vi "RecursiveNavigateHCC.vi"(9 "SearchingFor":string="body", 11 "data":string="<!DOCTYPE HTML PUBLIC \"-//IETF//DTD HTML//EN\">\r\n<HTML>\r\n<HEAD>\r\n<meta name=\"generator\" content=\"Microsoft&reg; HTML Help Workshop 4.1\">\r\n<!-- Sitemap 1.0 -->\r\n</head>\r\n<body>\r\n   <OBJECT type=\"text/site properties\">\r\n     <param name=\"Window Styles\" value=\"0x800025\">\r\n     <param name=\"comment\" value=\"title:Online Help\">\r\n     <param name=\"comment\" value=\"base:index.htm\">\r\n   </OBJECT>\r\n   <UL>\r\n      <LI><OBJECT type=\"text/sitemap\">\r\n            <param name=\"Name\" value=\"Main\">\r\n            <param name=\"Local\" value=\"main/main.html\">\r\n            <param name=\"ImageNumber\" value=\"2\">\r\n          </OBJECT>\r\n      <LI><OBJECT type=\"text/sitemap\">\r\n            <param name=\"Name\" value=\"Alarms\">\r\n            <param name=\"Local\" value=\"alarms/alarms.html\">\r\n            <param name=\"ImageNumber\" value=\"11\">\r\n          </OBJECT>\r\n      <LI><OBJECT type=\"text/sitemap\">\r\n            <param name=\"Name\" value=\"Calibration\">\r\n            <param name=\"Local\" value=\"calibration/calibration.html\">\r\n            <param name=\"ImageNumber\" value=\"11\">\r\n          </OBJECT>\r\n      <LI><OBJECT type=\"text/sitemap\">\r\n            <param name=\"Name\" value=\"Channel setting\">\r\n            <param name=\"Local\" value=\"channels%20setting/channel_setting.html\">\r\n            <param name=\"ImageNumber\" value=\"11\">\r\n          </OBJECT>\r\n      <LI><OBJECT type=\"text/sitemap\">\r\n            <param name=\"Name\" value=\"Create deltas\">\r\n            <param name=\"Local\" value=\"create%20delta/create_deltas.html\">\r\n            <param name=\"ImageNumber\" value=\"11\">\r\n          </OBJECT>\r\n      <LI><OBJECT type=\"text/sitemap\">\r\n            <param name=\"Name\" value=\"Criteria window\">\r\n            <param name=\"Local\" value=\"criteria/criteria_window.html\">\r\n            <param name=\"ImageNumber\" value=\"11\">\r\n          </OBJECT>\r\n      <LI><OBJECT type=\"text/sitemap\">\r\n            <param name=\"Name\" value=\"Filters\">\r\n            <param name=\"Local\" value=\"filters/filters.html\">\r\n          </OBJECT>\r\n      <UL>\r\n         <LI><OBJECT type=\"text/sitemap\">\r\n               <param name=\"Name\" value=\"Differential\">\r\n               <param name=\"Local\" value=\"filters/differential_filter.html\">\r\n               <param name=\"ImageNumber\" value=\"11\">\r\n             </OBJECT>\r\n         <LI><OBJECT type=\"text/sitemap\">\r\n               <param name=\"Name\" value=\"IIR-FIR\">\r\n               <param name=\"Local\" value=\"filters/iir_fir_filter.html\">\r\n               <param name=\"ImageNumber\" value=\"11\">\r\n             </OBJECT>\r\n         <LI><OBJECT type=\"text/sitemap\">\r\n               <param name=\"Name\" value=\"Median\">\r\n               <param name=\"Local\" value=\"filters/median_filter.html\">\r\n               <param name=\"ImageNumber\" value=\"11\">\r\n             </OBJECT>\r\n         <LI><OBJECT type=\"text/sitemap\">\r\n               <param name=\"Name\" value=\"Wavelet\">\r\n               <param name=\"Local\" value=\"filters/wavelet_filter.html\">\r\n               <param name=\"ImageNumber\" value=\"11\">\r\n             </OBJECT>\r\n      </UL>\r\n      <LI><OBJECT type=\"text/sitemap\">\r\n            <param name=\"Name\" value=\"Last defect window\">\r\n            <param name=\"Local\" value=\"last%20defect%20window/last_defect_window.html\">\r\n            <param name=\"ImageNumber\" value=\"11\">\r\n          </OBJECT>\r\n      <LI><OBJECT type=\"text/sitemap\">\r\n            <param name=\"Name\" value=\"Live view\">\r\n            <param name=\"Local\" value=\"live%20view/live_view.html\">\r\n            <param name=\"ImageNumber\" value=\"11\">\r\n          </OBJECT>\r\n      <LI><OBJECT type=\"text/sitemap\">\r\n            <param name=\"Name\" value=\"Oscilloscope\">\r\n            <param name=\"Local\" value=\"oscilloscope/oscilloscope.html\">\r\n            <param name=\"ImageNumber\" value=\"11\">\r\n          </OBJECT>\r\n      <LI><OBJECT type=\"text/sitemap\">\r\n            <param name=\"Name\" value=\"Record data\">\r\n            <param name=\"Local\" value=\"record%20data/record_data_window.html\">\r\n            <param name=\"ImageNumber\" value=\"11\">\r\n          </OBJECT>\r\n      <LI><OBJECT type=\"text/sitemap\">\r\n            <param name=\"Name\" value=\"Stripchart\">\r\n            <param name=\"Local\" value=\"stripchart%20Vpp/stripchart.html\">\r\n            <param name=\"ImageNumber\" value=\"11\">\r\n          </OBJECT>\r\n      <LI><OBJECT type=\"text/sitemap\">\r\n            <param name=\"Name\" value=\"System info\">\r\n            <param name=\"Local\" value=\"system%20info/system_info.html\">\r\n            <param name=\"ImageNumber\" value=\"11\">\r\n          </OBJECT>\r\n      <LI><OBJECT type=\"text/sitemap\">\r\n            <param name=\"Name\" value=\"System settings\">\r\n            <param name=\"Local\" value=\"system%20settings/system_settings.html\">\r\n            <param name=\"ImageNumber\" value=\"11\">\r\n          </OBJECT>\r\n      <LI><OBJECT type=\"text/sitemap\">\r\n            <param name=\"Name\" value=\"Vumeter\">\r\n            <param name=\"Local\" value=\"vumeter/vumeter.html\">\r\n            <param name=\"ImageNumber\" value=\"11\">\r\n          </OBJECT>\r\n      <LI><OBJECT type=\"text/sitemap\">\r\n            <param name=\"Name\" value=\"Wizard\">\r\n            <param name=\"Local\" value=\"wizard/wizard.html\">\r\n          </OBJECT>\r\n      <UL>\r\n         <LI><OBJECT type=\"text/sitemap\">\r\n               <param name=\"Name\" value=\"Step 1\">\r\n               <param name=\"Local\" value=\"wizard/wizard_step_1.html\">\r\n               <param name=\"ImageNumber\" value=\"11\">\r\n             </OBJECT>\r\n         <LI><OBJECT type=\"text/sitemap\">\r\n               <param name=\"Name\" value=\"Step 2\">\r\n               <param name=\"Local\" value=\"wizard/wizard_step_2.html\">\r\n               <param name=\"ImageNumber\" value=\"11\">\r\n             </OBJECT>\r\n         <LI><OBJECT type=\"text/sitemap\">\r\n               <param name=\"Name\" value=\"Step 3\">\r\n               <param name=\"Local\" value=\"wizard/wizard_step_3.html\">\r\n               <param name=\"ImageNumber\" value=\"11\">\r\n             </OBJECT>\r\n         <LI><OBJECT type=\"text/sitemap\">\r\n               <param name=\"Name\" value=\"Step 4\">\r\n               <param name=\"Local\" value=\"wizard/wizard_step_4.html\">\r\n               <param name=\"ImageNumber\" value=\"11\">\r\n             </OBJECT>\r\n         <LI><OBJECT type=\"text/sitemap\">\r\n               <param name=\"Name\" value=\"Step 5\">\r\n               <param name=\"Local\" value=\"wizard/wizard_step_5.html\">\r\n               <param name=\"ImageNumber\" value=\"11\">\r\n             </OBJECT>\r\n         <LI><OBJECT type=\"text/sitemap\">\r\n               <param name=\"Name\" value=\"Step 6\">\r\n               <param name=\"Local\" value=\"wizard/wizard_step_6.html\">\r\n               <param name=\"ImageNumber\" value=\"11\">\r\n             </OBJECT>\r\n      </UL>\r\n   </UL>\r\n</BODY>\r\n</HTML>\r\n") -> (1 "ItemTags":string[](array[string]), 2 "Ident":i32[](array[numeric]), 3 "ItemNames":string[](array[string]))   [LabVIEW 2016, in "Folder_Mgmt.lvclass"]
uses:
  Folder_Mgmt.lvclass
  <vilib>/regexp/Match Regular Expression.xnode
panel:
  in  "TestString":string="<!DOCTYPE HTML PUBLIC \"-//IETF//DTD HTML//EN\">\r\n<HTML>\r\n<HEAD>\r\n<meta name=\"generator\" content=\"Microsoft&reg; HTML Help Workshop 4.1\">\r\n<!-- Sitemap 1.0 -->\r\n</head>\r\n<body>\r\n   <OBJECT type=\"text/site properties\">\r\n     <param name=\"Window Styles\" value=\"0x800025\">\r\n     <param name=\"comment\" value=\"title:Online Help\">\r\n     <param name=\"comment\" value=\"base:index.htm\">\r\n   </OBJECT>\r\n   <UL>\r\n      <LI><OBJECT type=\"text/sitemap\">\r\n            <param name=\"Name\" value=\"Main\">\r\n            <param name=\"Local\" value=\"main/main.html\">\r\n            <param name=\"ImageNumber\" value=\"2\">\r\n          </OBJECT>\r\n      <LI><OBJECT type=\"text/sitemap\">\r\n            <param name=\"Name\" value=\"Alarms\">\r\n            <param name=\"Local\" value=\"alarms/alarms.html\">\r\n            <param name=\"ImageNumber\" value=\"11\">\r\n          </OBJECT>\r\n   </UL>\r\n</BODY>\r\n</HTML>\r\n"
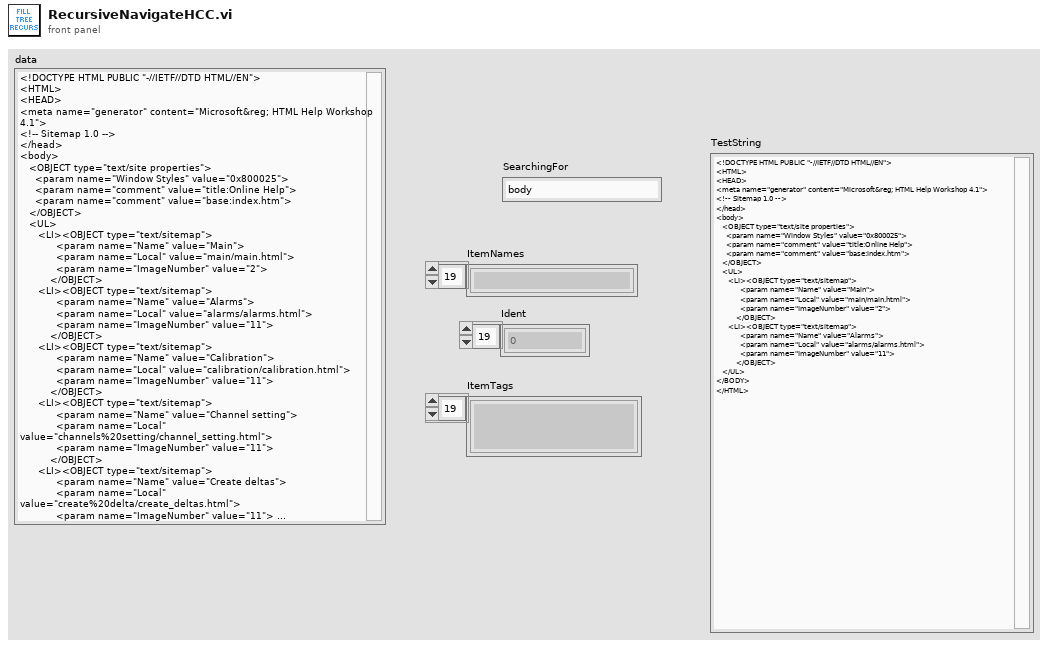
[diagram p1: front panel]
types:
  T1 = enum16{"Initialize", "Get All", "Add ItemName", "Add Ident", "Add Item Tag"}
  T2 = enum16{"Initialize", "Get All", "Add ItemName", "Add Ident", "Add Item Tag", "CurrIdentPlus", "CurrIdentMinus", "ResetFirstAcquired"}
  T3 = enum16{"Initialize", "Get All", "Add ItemName", "Add Ident", "Add Item Tag", "CurrIdentPlus", "CurrIdentMinus"}
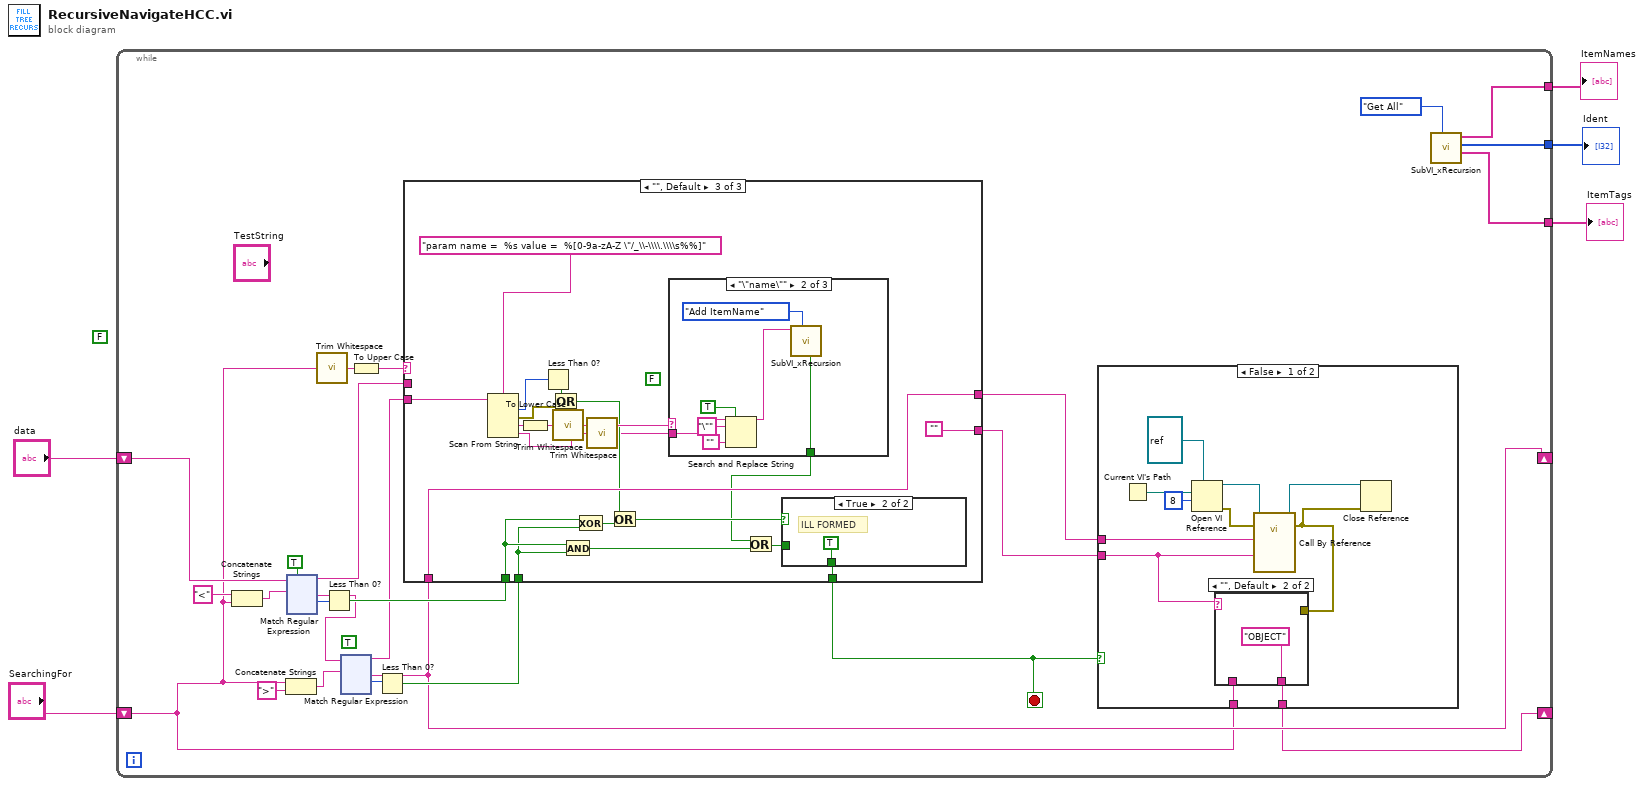
[diagram p0: block diagram]
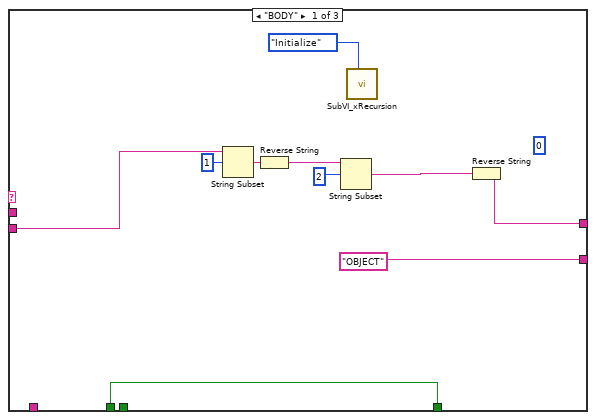
[diagram p2: hidden frame]
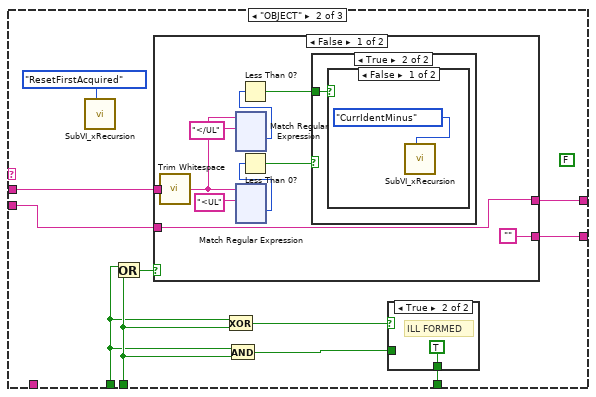
[diagram p3: hidden frame]
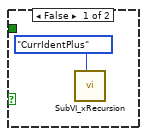
[diagram p4: hidden frame]
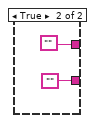
[diagram p6: hidden frame]
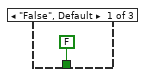
[diagram p8: hidden frame]
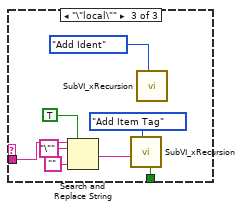
[diagram p9: hidden frame]
diagram:
  (unwired) FALSE
  n1 = while {
    shift-right: [w12] -> _
    shift-left: "data" -> [w26]
    shift-right: [w7] -> _
    shift-left: "SearchingFor" -> [w6]
    tunnel: [w10] -> w3
    tunnel: [w9] -> w2
    tunnel: [w8] -> w1
    stop <- w15 stop-if-true
    (unwired) TRUE ("ignore case? (F)")
    n2 = Concatenate Strings("<" ("string"), w6) -> (w30:string)
    n3 = Concatenate Strings(w6, ">" ("string")) -> (w23:string)
    n4 = xnode "Match Regular Expression"("input string"=w26, "regular expression"=w30, "ignore case? (F)"=TRUE) -> ("before match"=w17:string, "after match"=w22:string, "offset past match"=w27:i32)  [unwired: 3 in, 2 out]
    n5 = call <vilib>:"Trim Whitespace.vi"("string"=w6) -> ("trimmed string"=w14:string)  [unwired: 1 in]
    n6 = Less Than 0?(x=w27) -> (x < 0?=w24:bool)
    n7 = xnode "Match Regular Expression"("input string"=w22, "regular expression"=w23) -> ("before match"=w21:string, "after match"=w12:string, "offset past match"=w20:i32)  [unwired: 4 in, 2 out]
    n8 = To Upper Case(1:w14) -> (0:w13:string)
    n9 = Less Than 0?(x=w20) -> (x < 0?=w19:bool)
    n10 = case shown="\"\", Default" w13 {
      tunnel: [w146 w159 w421] -> w25
      tunnel: w21 -> [w152 w156 w428]
      tunnel: w24 -> [w153 w160 w420]
      tunnel: ["OBJECT" w158 ""] -> w16
      tunnel: w19 -> [_ w161 w419]
      tunnel: [w153 w163 w429] -> w15
      tunnel: w17 -> [_ w157 _]
      tunnel: w12 -> [_ _ w421]
      frame "BODY" {
        (unwired) 0
        n11 = String Subset(string=w152, offset (0)=1) -> (substring=w150:string)  [unwired: 1 in]
        n12 = Reverse String(1:w150) -> (0:w148:string)
        n13 = String Subset(string=w148, offset (0)=2) -> (substring=w147:string)  [unwired: 1 in]
        n14 = call "SubVI_xRecursion.vi"("Enum"=T1."Initialize") -> ()  [unwired: 7 in, 4 out]
        n15 = Reverse String(1:w147) -> (0:w146:string)
      }
      frame "OBJECT" {
        (unwired) FALSE
        n16 = call "SubVI_xRecursion.vi"("Enum"=T2."ResetFirstAcquired") -> ()  [unwired: 7 in, 4 out]
        n17 = Or(x=w160, y=w161) -> (x .or. y?=w162:bool)
        n18 = case shown="False" w162 {
          tunnel: [w173 ""] -> w159
          tunnel: ["" ""] -> w158
          tunnel: w157 -> [w169 _]
          tunnel: w156 -> [w173 _]
          frame False {
            n19 = call <vilib>:"Trim Whitespace.vi"("string"=w169) -> ("trimmed string"=w166:string)  [unwired: 1 in]
            n20 = xnode "Match Regular Expression"("input string"=w166, "regular expression"="</UL" ("string")) -> ("offset past match"=w170:i32)  [unwired: 4 in, 4 out]
            n21 = xnode "Match Regular Expression"("input string"=w166, "regular expression"="<UL" ("string")) -> ("offset past match"=w174:i32)  [unwired: 4 in, 4 out]
            n22 = Less Than 0?(x=w170) -> (x < 0?=w167:bool)
            n23 = Less Than 0?(x=w174) -> (x < 0?=w171:bool)
            n24 = case shown="True" w171 {
              tunnel: w167 -> [_ w291]
              frame False {
                n25 = call "SubVI_xRecursion.vi"("Enum"=T3."CurrIdentPlus") -> ()  [unwired: 7 in, 4 out]
              }
              frame True {
                n26 = case shown="False" w291 {
                  frame False {
                    n27 = call "SubVI_xRecursion.vi"("Enum"=T3."CurrIdentMinus") -> ()  [unwired: 7 in, 4 out]
                  }
                  frame True {
                  }
                }
              }
            }
          }
          frame True {
          }
        }
        n28 = Exclusive Or(1:w161, 2:w160) -> (0:w165:bool)
        n29 = And(x=w160, y=w161) -> (x .and. y?=w164:bool)
        n30 = case shown="True" w165 {
          tunnel: w164 -> [w409 _]
          tunnel: [w409 TRUE] -> w163
          frame False {
            # "FINISH"
          }
          frame True {
            # "ILL FORMED"
          }
        }
      }
      frame "", Default {
        (unwired) FALSE ("x")
        n31 = Scan From String(format string="param name =  %s value =  %[0-9a-zA-Z \"/_\\-\\\\.\\\\s%%]", input string=w428) -> (offset past scan=w427:u32, error out=w423:errorcluster, output 1=w425:string, output 2=w412:string)  [unwired: 4 in, 1 out]
        n32 = To Lower Case(string=w425) -> (all lower case string=w424:string)
        n33 = Less Than 0?(x=w427) -> (x < 0?=w426:bool)
        n34 = Or(x=w426, y=w423) -> (x .or. y?=w415:bool)
        n35 = call <vilib>:"Trim Whitespace.vi"("string"=w424) -> ("trimmed string"=w422:string)  [unwired: 1 in]
        n36 = And(x=w420, y=w419) -> (x .and. y?=w417:bool)
        n37 = Exclusive Or(1:w419, 2:w420) -> (0:w430:bool)
        n38 = call <vilib>:"Trim Whitespace.vi"("string"=w412) -> ("trimmed string"=w413:string)  [unwired: 1 in]
        n39 = Or(x=w415, y=w430) -> (x .or. y?=w416:bool)
        n40 = case shown="\"\\\"name\\\"\"" w422 {
          tunnel: w413 -> [_ w439 w445]
          tunnel: [FALSE w434 w440] -> w414
          frame "False", Default {
          }
          frame "\"name\"" {
            n41 = Search and Replace String(replace all?=TRUE ("replace all? (F)"), input string=w439, search string="\"", replace string="") -> (result string=w433:string)  [unwired: 4 in, 3 out]
            n42 = call "SubVI_xRecursion.vi"("Enum"=T1."Add ItemName", "ItemName"=w433) -> ("FirstAcquired"=w434:bool)  [unwired: 6 in, 3 out]
          }
          frame "\"local\"" {
            n43 = Search and Replace String(replace all?=TRUE ("replace all? (F)"), input string=w445, search string="\"", replace string="") -> (result string=w442:string)  [unwired: 4 in, 3 out]
            n44 = call "SubVI_xRecursion.vi"("Enum"=T1."Add Item Tag", "ItemTag"=w442) -> ("FirstAcquired"=w440:bool)  [unwired: 6 in, 3 out]
            n45 = call "SubVI_xRecursion.vi"("Enum"=T1."Add Ident") -> ()  [unwired: 7 in, 4 out]
          }
        }
        n46 = Or(x=w414, y=w417) -> (x .or. y?=w418:bool)
        n47 = case shown="True" w416 {
          tunnel: w418 -> [w448 _]
          tunnel: [w448 TRUE] -> w429
          frame False {
            # "FINISH"
          }
          frame True {
            # "ILL FORMED"
          }
        }
      }
    }
    n48 = case shown="False" w15 {
      tunnel: w25 -> [w568 _]
      tunnel: w16 -> [w564 _]
      tunnel: [w566 w577] -> w7
      tunnel: w6 -> [w567 w577]
      frame False {
        n49 = Current VI's Path() -> (path=w574:path)
        n50 = Open VI Reference(type specifier VI Refnum (for type only)=refnum<vi> refnum, vi path=w574, options=8) -> (vi reference=w571:refnum<vi>, error out=w570:errorcluster)  [unwired: 3 in]
        n51 = call-by-ref "?"(reference=w571, error in=w570, "SearchingFor"=w564, "data"=w568) -> (reference out=w569:refnum<vi>, error out=w565:errorcluster)  [unwired: 7 in, 3 out]
        n52 = case shown="\"\", Default" w564 {
          tunnel: [w575 "OBJECT"] -> w566
          tunnel: w567 -> [w575 _]
          tunnel: w565 -> [_ _]
          frame "OBJECT" {
          }
          frame "", Default {
          }
        }
        n53 = Close Reference(reference=w569, error in (no error)=w565) -> ()  [unwired: 1 out]
      }
      frame True {
      }
    }
    n54 = call "SubVI_xRecursion.vi"("Enum"=T1."Get All") -> ("ItemTags 2"=w8:string[], "Ident 2"=w9:i32[], "ItemNames 2"=w10:string[])  [unwired: 7 in, 1 out]
  }
  "ItemNames" <- w3
  "Ident" <- w2
  "ItemTags" <- w1
